vi "backup_from_wall.vi"(11 "NXT":T1={"Hardware"="NXT", "Flattened String"=""}) -> (3 "NXT2":T1 caption="NXT")   [LabVIEW 2012]
uses:
  <vilib>/NXT/Subs/LVHSConnector.ctl
  <vilib>/NXT/Subs/MotorOutput.ctl
  <vilib>/NXT/Dual Mode Library/Motors/MotorOn.vi
  <vilib>/NXT/Dual Mode Library/Motors/MotorBrake.vi
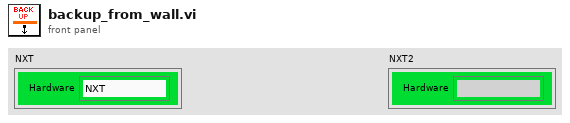
[diagram p1: front panel]
types:
  T1 = typedef "LVHSConnector.ctl" = cluster{"Hardware":string, "Flattened String":string}
  T2 = typedef "MotorOutput.ctl" = u8
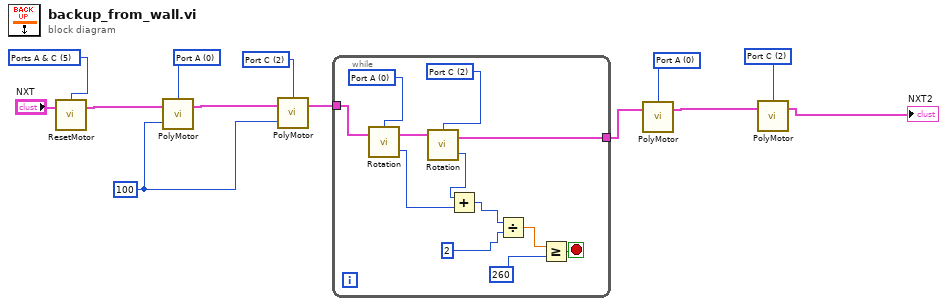
[diagram p0: block diagram]
diagram:
  w6 = T2 2 items=["Port A"=0, "Port B"=1, "Port C"=2, "Ports A & B"=4, "Ports A & C"=5, "Ports B & C"=6, "All Ports"=3] ("Output Port (All Ports)")
  w4 = T2 0 items=["Port A"=0, "Port B"=1, "Port C"=2, "Ports A & B"=4, "Ports A & C"=5, "Ports B & C"=6, "All Ports"=3] ("Output Port (All Ports)")
  w8 = 100
  w10 = T2 2 items=["Port A"=0, "Port B"=1, "Port C"=2, "Ports A & B"=4, "Ports A & C"=5, "Ports B & C"=6, "All Ports"=3] ("Output Port (All Ports)")
  w12 = T2 0 items=["Port A"=0, "Port B"=1, "Port C"=2, "Ports A & B"=4, "Ports A & C"=5, "Ports B & C"=6, "All Ports"=3] ("Output Port (All Ports)")
  w13 = T2 5 items=["Port A"=0, "Port B"=1, "Port C"=2, "Ports A & B"=4, "Ports A & C"=5, "Ports B & C"=6, "All Ports"=3] ("Output Port (All Ports)")
  n1 = call <vilib>:"ResetMotor.vi"("NXT"="NXT", "Port (All Ports)"=w13) -> ("NXT"=w7:T1)  [unwired: 2 in]
  n2 = call-poly <vilib>:"PolyMotor.vi"("Power (75)"=w8, "NXT"=w7, "Output Port (All Ports)"=w12) -> ("NXT"=w11:T1)  [unwired: 1 in]
  n3 = call-poly <vilib>:"PolyMotor.vi"("Power (75)"=w8, "NXT"=w11, "Output Port (All Ports)"=w10) -> ("NXT"=w9:T1)  [unwired: 1 in]
  n4 = while {
    tunnel: w9 -> [w23]
    tunnel: [w22] -> w3
    stop <- w15 stop-if-true
    w21 = T2 2 items=["Port A"=0, "Port B"=1, "Port C"=2, "Ports A & B"=4, "Ports A & C"=5, "Ports B & C"=6, "All Ports"=3] ("Output Port (All Ports)")
    w24 = T2 0 items=["Port A"=0, "Port B"=1, "Port C"=2, "Ports A & B"=4, "Ports A & C"=5, "Ports B & C"=6, "All Ports"=3] ("Output Port (All Ports)")
    n5 = call <vilib>:"Rotation.vi"("NXT"=w23, "Port (Port A)"=w24) -> ("Angle of Rotation"=w18:i32, "NXT"=w25:T1)  [unwired: 1 in]
    n6 = call <vilib>:"Rotation.vi"("NXT"=w25, "Port (Port A)"=w21) -> ("Angle of Rotation"=w17:i32, "NXT"=w22:T1)  [unwired: 1 in]
    n7 = Add(x=w17, y=w18) -> (x+y=w19:i32)
    n8 = Divide(x=w19, y=2) -> (x/y=w16:dbl)
    n9 = Greater Or Equal?(x=w16, y=260) -> (x >= y?=w15:bool)
  }
  n10 = call-poly <vilib>:"PolyMotor.vi"("NXT"=w3, "Port (All Ports)"=w4) -> ("NXT"=w5:T1)  [unwired: 2 in]
  n11 = call-poly <vilib>:"PolyMotor.vi"("NXT"=w5, "Port (All Ports)"=w6) -> ("NXT"=→"NXT2":T1)  [unwired: 2 in]
